vi "Constants.vi"() -> ()   [LabVIEW 2014, in "SLSC configuration Shared.lvlib"]
uses:
  SLSC configuration Shared.lvlib
panel:
  in  "Tab Control":T1(tab)=enum."Constants"
  in  "GUID.UEGO channel":string="084a2bde-6980-4a25-8dc9-17562dca28ac"
  in  "GUID.DIO channel":string="68b1edbf-44ca-4db8-a110-9c4878466134"
  in  "GUID.LEDs channel":string="3daa6cb5-932b-450d-8512-df794f896397"
  in  "GUID.LEDs card":string="855718a2-01fd-4326-a70b-94b32735622c"
  in  "GUID.Current Sense channel":string="96dbb118-ce34-4cee-8d88-4cdf2e4dc3eb"
  in  "GUID.Current Sense card":string="22a74749-cb4a-4d08-9a57-d9f882501be9"
  in  "GUID.SLSC Disabled":string="8eabe605-99e1-4ccd-8dc0-f89f19004ff1"
  in  "GUID.UEGO card":string="ca3bbe61-0f5e-4312-bf6e-b2e5f37b2ab6"
  in  "GUID.WSS channel":string="b1057e8f-4024-44e6-964c-b22fb6b0c38d"
  in  "GUID.WSS card":string="f4221155-5f1c-4cea-ae03-1d5c2b71466f"
  in  "GUID.Battery Switch channel":string="1c2c1f1a-3a58-495a-bf7b-e933ed2669ef"
  in  "GUID.Battery Switch card":string="088b733f-dcb6-43c3-89b9-85f1a5efe81e"
  in  "GUID.Resistor Channel":string="c1df0500-e9fe-462d-a67f-7c6056707f28"
  in  "GUID.Resistor Card":string="8c9eb810-a56f-48f6-b7a1-40928e14985f"
  in  "GUID.FIU line":string="419d9b57-9547-4c03-8a6e-b71d44e1efd6"
  in  "GUID.DIO card":string="7fc51c5c-63e7-4d2e-8e21-24b5aba9210e"
  in  "GUID.FIU card":string="8a7a6458-bb89-4ca3-ad7b-82e230caa836"
  in  "GUID.SLSC":string="1669feb8-c7a5-4ea6-863a-145b2f30e50b"
  in  "duplicate slot":string="The card slot you selected is already in use. Please select a different slot, or delete the card that has already been added in this slot"
  in  "duplicate name":string="The name you selected is already in use. Please select a different name."
  in  "DIO.Logic Threshold #":string="DIO.Logic Threshold #"
  in  "DIO.Line Config 3":string="DIO Line Config 3"
  in  "DIO.Line Config 2":string="DIO Line Config 2"
  in  "DIO.Line Config 1":string="DIO Line Config 1"
  in  "DIO.Line Config 0":string="DIO Line Config 0"
  in  "DIO.Logic Threshold 3":string="Logic Threshold 3"
  in  "DIO.Logic Threshold 2":string="Logic Threshold 2"
  in  "DIO.Logic Threshold 1":string="Logic Threshold 1"
  in  "DIO.Logic Threshold 0":string="Logic Threshold 0"
  in  "DIO Config":string="DIO Config"
  in  "Generic.Max # of Racks":string="Max # of Racks"
  in  "Generic.SLSC FPGA Settings":string="SLSC FPGA Settings"
  in  "Generic.FIFO Name":string="FIFO Name"
  in  "Generic.Device Settings":string="Device Settings"
  in  "Generic.RIO Dev Address":string="RIO Dev Address"
  in  "Generic.Load Delay":string="Load Delay"
  in  "Generic.Sample Rate":string="Sample Rate"
  in  "Generic.Divide Value":string="Divide Value"
  in  "Generic.Slot #":string="Slot #"
  in  "Generic.Rack #":string="Rack #"
  in  "Generic.Bitfile Path":string="BItfile Path"
  in  "FPGA Name":string="FPGA Name"
  in  "Compiled Info":string="Compiled Info"
  in  "Card Postion":string="Card Position"
  in  "Constants.UEGO Chip Address":u8 format="%02b"
  in  "Constants.# of UEGO Channels":u8=4
  in  "Constants.# of DIO Channels":u8=4
  in  "Constants.DIO Default Threshold":u16=50
  in  "Constants.LED Chip Address":u8 format="%02b"
  in  "Constants.# of LEDs":u8=8
  in  "Constants.LEDs":string="LEDs"
  in  "Constants.# of Curr Channels":u8=16
  in  "Constants.Curr Chip Address":u8 format="%02b"
  in  "Constants.Current Sense":string="Current Sense"
  in  "Constants.go name":string="slsc.go"
  in  "Constants.UEGO":string="UEGO"
  in  "Constants.Resistor Chip Addresses":u8[](array[numeric])=[0, 1, 2, 3, 4, 5, 6, 7] format="%.0b"
  in  "Constants.# of Resistor Channels":u8=8
  in  "Constants.Resistor":string="Resistor"
  in  "Constants.WSS Chip Address":u8 format="%02b"
  in  "Constants.# of WSS Channels":u8=4
  in  "Constants.WSS":string="WSS"
  in  "Constants.BATT Chip Address":u8 format="%02b"
  in  "Constants.BATT":string="BATT"
  in  "Constants.# of BATT Switches":u8=3
  in  "Constants.RT base path":path=path "c:/ni-rt/NIVeriStand/Custom Devices/SLSC"
  in  "Constants.Invalid bitfile":string="Invalid bitfile"
  in  "Constants.FPGA FIFO Name":string="slsc.FIFO Name."
  in  "Constants.FPGA # of racks":string="slsc.# of Racks."
  in  "Constants.# of FIU Channels per Chip":u8=4
  in  "Constants.FIU Chip Addresses":u8[](array[numeric])=[0, 1] format="%02b"
  in  "Constants.DIO Chip Addresses":u8[](array[numeric])=[0, 1, 2, 3] format="%02b"
  in  "Constants.# of Slots":u8=16
  in  "Constants.DIO":string="DIO"
  in  "Constants.# of FIU Channels":u8=8
  in  "Constants.FIU":string="FIU"
  in  "Constants.Sample Rate":string="Sample Rate (S/s)"
  in  "Constants.SPI PHY Settings":string="SPI PHY Settings"
  in  "Constants.DMA FIFO":string="SPI CMD FIFO"
  in  "Constants.UEGO Calibration Complete Name":string="UEGOcalibration.Complete?"
  in  "FIU.Fault #":string="Fault #"
  in  "LEDs.LED #":string="LEDs.LED #"
  in  "BATT.Switch #":string="Switch #"
  in  "WSS.Channel #":string="WSS.Channel #"
  in  "Resistor.Channel #":string="Resistor.Channel #"
  in  "UEGO.Channel #":string="UEGO.Channel #"
  in  "UEGO.FPGA Item Name":string="UEGO.FPGA Item Name"
  in  "UEGO.Compiled Settings":string="UEGO.Compiled Settings"
  in  "UEGO.HW Settling Time":string="UEGO.HW Settling Time"
  in  "UEGO.Calibration Time":string="UEGO.Calibration Time"
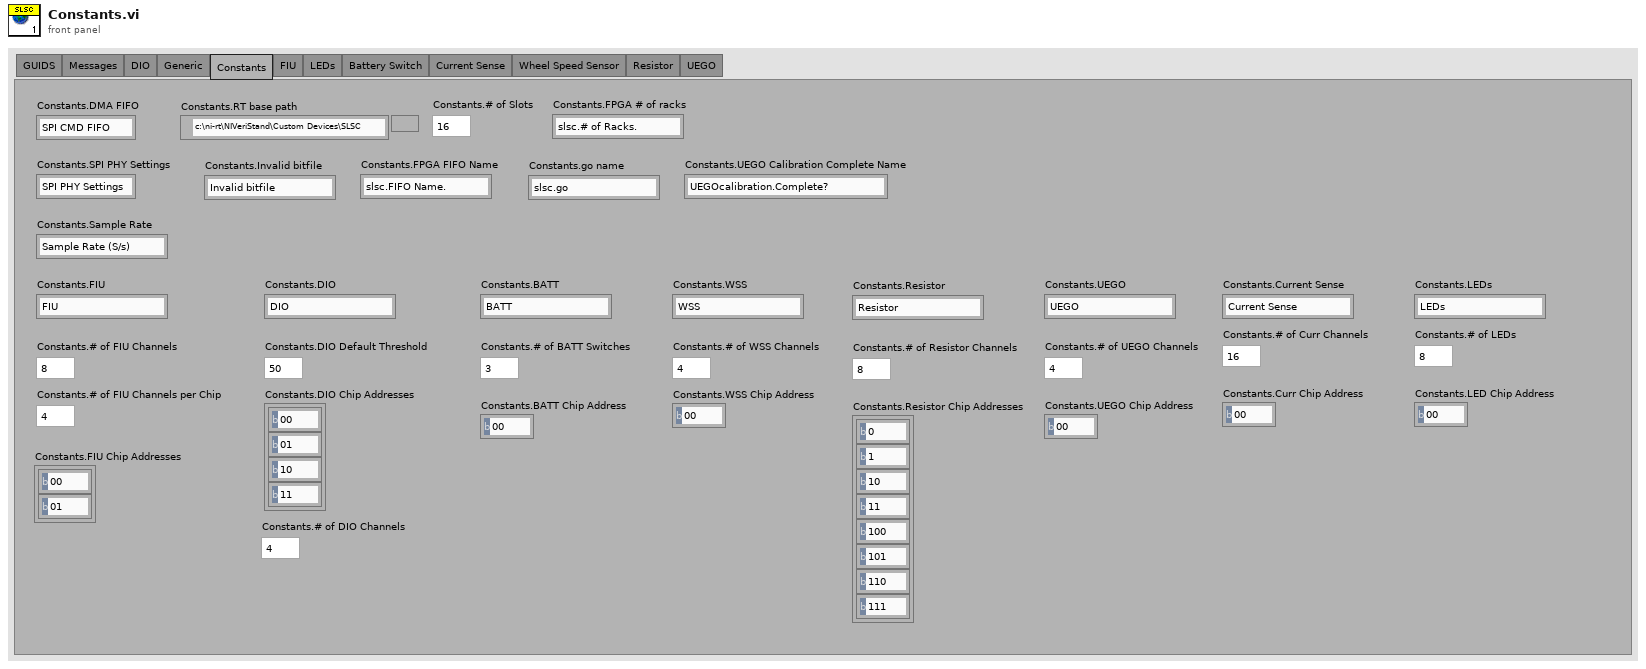
[diagram p1: front panel]
types:
  T1 = enum32{"GUIDS", "Messages", "DIO", "Generic", "Constants", "FIU", "LEDs", "Battery Switch", "Current Sense", "Wheel Speed Sensor", "Resistor", "UEGO"}
diagram:
